vi "Manage Inputs.vi"(6 "Discard action? (F)":bool, 7 "Communication in":refnum<class "Communication.lvclass">, 11 "Game Board in":refnum<class "Game Board.lvclass">) -> (3 "Game Board out":refnum<class "Game Board.lvclass">)   [LabVIEW 2024, in "Game Board.lvclass"]
doc: "MIT Licence\nCopyright (c) 2024 David Grollier"
uses:
  Game Board.lvclass
  Communication/Communication.lvclass
  Communication/Communication.lvclass/Communication.ctl
  Game Board.lvclass/Game Board.ctl
  Action Command.ctl
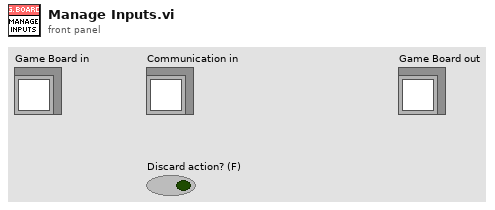
[diagram p1: front panel]
types:
  T1 = typedef "Game Board.lvclass/Action Command.ctl" = cluster{"Boost":bool}
  T2 = typedef "Game Board.lvclass/Player command.ctl" = cluster{"Direction":cluster{dbl, dbl}, "Velocity":dbl}
  T3 = typedef "Xbox Controller.lvclass/Action commands.ctl" = cluster{"Boost":bool}
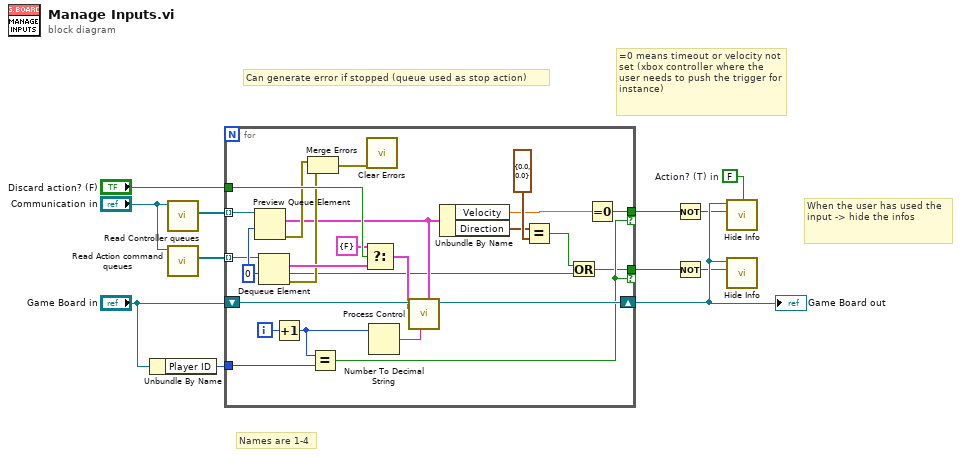
[diagram p0: block diagram]
diagram:
  w1 = FALSE  # Action? (T) in
  # "=0 means timeout or velocity not set (xbox controller where the user needs to push the trigger for instance)"
  # "Can generate error if stopped (queue used as stop action)"
  # "When the user has used the input -> hide the infos"
  # "Names are 1-4"
  n1 = Unbundle By Name("Game Board in") -> ("Player ID"=w7:i64)
  n2 = call "Read Controller queues.vi"("Communication in"="Communication in") -> ("State command queues"=w10:refnum<queue>[])  [unwired: 10 in]
  n3 = call "Read Action command queues.vi"("Communication in"="Communication in") -> ("Action command queues out"=w11:refnum<queue>[])  [unwired: 10 in]
  n4 = for {
    shift-right: [w36] -> w4
    shift-left: "Game Board in" -> [w37]
    tunnel: w10 -> [w34] mode=indexing
    tunnel: w11 -> [w33] mode=indexing
    tunnel: "Discard action? (F)" -> [w30]
    tunnel: w7 -> [w25]
    tunnel: [w20] -> w6 if=w24
    tunnel: [w13] -> w5 if=w24
    i -> [w32]
    w35 = 0 ("timeout in ms (-1)")
    n5 = Preview Queue Element(queue=w34, timeout in ms (-1)=w35) -> (element=w18:T2, error out=w23:errorcluster)  [unwired: 1 in, 2 out]
    n6 = Dequeue Element(queue=w33, timeout in ms (-1)=w35) -> (element=w29:T3, timed out?=w15:bool, error out=w22:errorcluster)  [unwired: 1 in, 1 out]
    n7 = Increment(x=w32) -> (x+1=w26:i32)
    n8 = Merge Errors(w23, w22) -> (w21:errorcluster)
    n9 = Equal?(x=w26, y=w25) -> (x = y?=w24:bool)
    n10 = Select(t=T1 {"Boost"=FALSE}, s=w30, f=w29) -> (s? t:f=w27:T3)
    n11 = call <vilib>:"Clear Errors.vi"("error in (no error)"=w21) -> ()  [unwired: 5 in, 2 out]
    n12 = Number To Decimal String(number=w26) -> (decimal integer string=w31:string)  [unwired: 1 in]
    n13 = call "Process Control.vi"("State in"=w18, "Name in"=w31, "Action in"=w27, "Game Board in"=w37) -> ("Game Board out"=w36:refnum<class "Game Board.lvclass">)  [unwired: 7 in]
    n14 = Unbundle By Name(w18) -> ("Velocity"=w16:dbl, "Direction"=w17:cluster{dbl, dbl})
    n15 = Equal?(x=w17, y=cluster{dbl, dbl} {0.0, 0.0} ("Direction")) -> (x = y?=w14:bool)
    n16 = Or(x=w14, y=w15) -> (x .or. y?=w13:bool)
    n17 = Equal To 0?(x=w16) -> (x = 0?=w20:bool)
  }
  "Game Board out" <- w4
  n18 = Not(x=w6) -> (.not. x?=w3:bool)
  n19 = Not(x=w5) -> (.not. x?=w2:bool)
  n20 = call "Hide Info.vi"("Action? (T) in"=w1, "Hide in"=w3, "Game Board in"=w4) -> ()  [unwired: 9 in]
  n21 = call "Hide Info.vi"("Hide in"=w2, "Game Board in"=w4) -> ()  [unwired: 10 in]
